vi "Eurotherm 35xx Series Process Value Monitoring.vi"() -> ()   [LabVIEW 2014]
doc: "This example demonstrates process value monitoring only.\n\nNote:\nEnter correct Resource Descriptor and Device Address into front-panel controls before you run this VI!\nBefore start this VI must be controller configuration ready and controller must run."
uses:
  <instrlib>/Eurotherm 35xx Series/Eurotherm 35xx Series.lvlib
panel:
  in  "stop":bool
  out "Process Value - Chart":i16(graph)
  out "Process Value":i16
  in  "Unit Address (1)":u8=1
  in  "VISA resource name":refnum<visa-resource-name>
  in  "Acknowledge All Alarms":bool
  out "ALARM !":bool
  # "(c) 2005-2010 NATIONAL INSTRUMENTS.  ALL RIGHTS RESERVED."
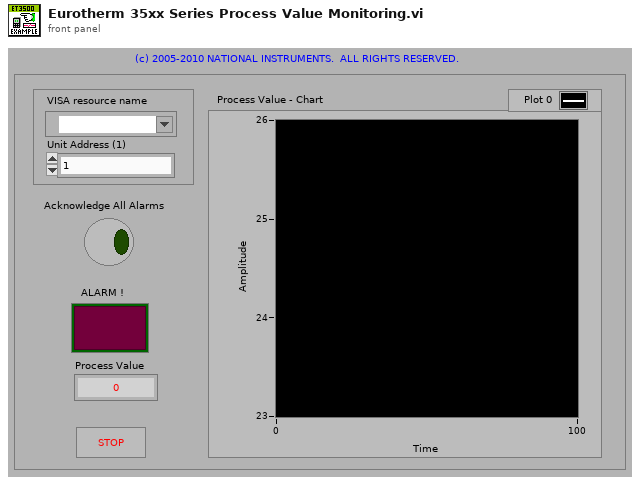
[diagram p1: front panel]
types:
  T1 = cluster{"Baud Rate (19200)":u32, "Parity (0: None)":u16, "Break Length (0)":u16}
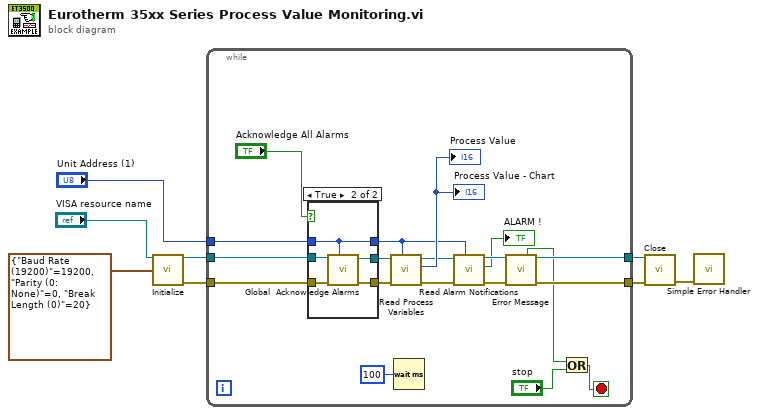
[diagram p0: block diagram]
diagram:
  n1 = call <instrlib>:"Initialize.vi"("VISA resource name"="VISA resource name", "Serial Configuration"=T1 {"Baud Rate (19200)"=19200, "Parity (0: None)"=0, "Break Length (0)"=20}) -> ("VISA resource name out"=w3:refnum<visa-resource-name>, "error out"=w2:errorcluster)  [unwired: 12 in]
  n2 = while {
    tunnel: w3 -> [w10]
    tunnel: w2 -> [w9]
    tunnel: "Unit Address (1)" -> [w11]
    tunnel: [w25] -> w5
    tunnel: [w24] -> w6
    stop <- w21 stop-if-true
    n3 = case shown="True" "Acknowledge All Alarms" {
      tunnel: w10 -> [w29 w35]
      tunnel: w9 -> [w28 w34]
      tunnel: [w29 w33] -> w13
      tunnel: [w28 w32] -> w12
      tunnel: w11 -> [w30 w31]
      tunnel: [w30 w31] -> w14
      frame False {
      }
      frame True {
        n4 = call <instrlib>:"Global  Acknowledge Alarms.vi"("Unit Address (1)"=w31, "error in (no error)"=w34, "VISA resource name"=w35) -> ("error out"=w32:errorcluster, "VISA resource name out"=w33:refnum<visa-resource-name>)  [unwired: 7 in]
      }
    }
    n5 = call <instrlib>:"Read Process Variables.vi"("Unit Address (1)"=w14, "error in (no error)"=w12, "VISA resource name"=w13) -> ("error out"=w15:errorcluster, "Process Value"=→"Process Value" →"Process Value - Chart":i16, "VISA resource name out"=w16:refnum<visa-resource-name>)  [unwired: 5 in, 1 out]
    n6 = Wait (ms)(milliseconds to wait=u32 100) -> ()  [unwired: 1 out]
    n7 = call <instrlib>:"Read Alarm Notifications.vi"("Unit Address (1)"=w14, "error in (no error)"=w15, "VISA resource name"=w16) -> ("error out"=w26:errorcluster, "New Alarm"=→"ALARM !":bool, "VISA resource name out"=w27:refnum<visa-resource-name>)  [unwired: 5 in, 1 out]
    n8 = call <instrlib>:"Error Message.vi"("VISA resource name"=w27, "error in (no error)"=w26) -> ("Status"=w19:bool, "VISA resource name out"=w25:refnum<visa-resource-name>, "error out"=w24:errorcluster)  [unwired: 9 in, 2 out]
    n9 = Or(x=w19, y="stop") -> (x .or. y?=w21:bool)
  }
  n10 = call <instrlib>:"Close.vi"("VISA resource name"=w5, "error in (no error)"=w6) -> ("error out"=w1:errorcluster)  [unwired: 13 in]
  n11 = call <vilib>:"Simple Error Handler.vi"("error in (no error)"=w1) -> ()  [unwired: 4 in, 5 out]
